vi "Full DMM Scan PRD 32 - 2 SCANs.vi"() -> ()   [LabVIEW 2021]
uses:
  DMM SCAN PRD 32V-16C/Typedefs/Scan configuration.ctl
  <instrlib>/niDMM/nidmm.llb/niDMM Resolution in Digits.ctl
  DMM SCAN PRD 32V-16C/Typedefs/Formatted measurement.ctl
  DMM SCAN PRD 32V-16C/Typedefs/Measurement values.ctl
  DMM Mixed Measurements/DMM Mixed Meas Typedefs/DMM Execution Settings.ctl
  DMM SCAN PRD 32V-16C/Typedefs/Scan Resource Names.ctl
  <instrlib>/niDMM/nidmm.llb/niDMM Powerline Frequency.ctl
  DMM SCAN PRD 32V-16C/Typedefs/Topology.ctl
  <instrlib>/niSwitch/niSwitch.llb/niSwitch Topologies.ctl
  DMM SCAN PRD 32V-16C/Typedefs/Switches Characteristics.ctl
  Static Digital Path Generation/Typedefs/Module Characteristics.ctl
  DMM SCAN PRD 32V-16C/DMM_Scan PXI RLY Driver 32V-16C.lvlib
  DMM Mixed Measurements/DMM_Mixed Measurement.lvlib
  Static Digital Path Generation/Switch_Static Digital Path Generation.lvlib
panel:
  out "Formatted Measurements 2":T1[](array[typedef])=[{"Channel"="ch1", "Switch Time"=0.03192880000005971, "Formatted Measurement"="97.3557mV (dc)", "Out of Range"=FALSE}, {"Channel"="ch32", "Switch Time"=0.040970100000095044, "Formatted Measurement"="9.43379uA (dc)", "Out of Range"=FALSE}, {"Channel"="ch0", "Switch Time"=0.030952699999943434, "Formatted Measurement"="9.89506V (dc)", "Out of Range"=FALSE}] {"Switch Time" format="%#_3p"}
  in  "Scan configuration 2":T2[](array[typedef])=[{"Channel"="ch1", "Resolution in Digits"=5.5, "Range and Function"=enum."DC 100 mV"}, {"Channel"="ch32", "Resolution in Digits"=5.5, "Range and Function"=enum."DC 10 uA"}, {"Channel"="ch0", "Resolution in Digits"=5.5, "Range and Function"=enum."DC 10 V"}] {"Resolution in Digits" items=["3 1/2"=3.5, "4 1/2"=4.5, "5 1/2"=5.5, "6 1/2"=6.5, "7 1/2"=7.5]}
  out "Total Scan Time (s) 2":dbl=0.10385570000016742 format="%#.3p"
  out "Switches Characteristics":T4
  in  "error in":errorcluster
  in  "Relays Debounce Time (ms)":u32=5
  in  "Close all Shunts?":bool=TRUE
  in  "Topology":T6={"MUX Topology Name"="2567/Independent"}
  in  "Powerline Frequency":T8=enum."50 Hz"
  in  "Scan Resources Names":T9={"DMM Resource Name"="DMM_4065", "MUX and Shunt Resource Name"="MUX_2567"}
  out "Total Scan Time (s)":dbl=0.22173839999982192 format="%#.3p"
  out "Execution Settings":T10[](array[typedef])=[{"Absolute\nResolution"=-1e-05, "Input Resistance\n(Ohm)"=10000000.0, "Digits\nResolution"=5.5, "Range"=-1.0, "Minimum\nFrequency (Hz)"=20.0, "Aperture\nTime (s)"=0.003333333333333333, "Auto Range\nValue"=10.0, "Settle\nTime (s)"=-1.0, "Function"=1}, {"Absolute\nResolution"=-1e-05, "Input Resistance\n(Ohm)"=10000000.0, "Digits\nResolution"=5.5, "Range"=-1.0, "Minimum\nFrequency (Hz)"=20.0, "Aperture\nTime (s)"=0.003333333333333333, "Auto Range\nValue"=0.1, "Settle\nTime (s)"=-1.0, "Function"=1}, {"Absolute\nResolution"=-1e-05, "Input Resistance\n(Ohm)"=-1.0, "Digits\nResolution"=5.5, "Range"=-1.0, "Minimum\nFrequency (Hz)"=20.0, "Aperture\nTime (s)"=0.003333333333333333, "Auto Range\nValue"=0.01, "Settle\nTime (s)"=-1.0, "Function"=3}] {"Function" items=["DC Volts"=1, "AC Volts"=2, "DC Current"=3, "AC Current"=4, "2-Wire Resistance"=5, "4-Wire Resistance"=101, "Frequency"=104, "Period"=105, "AC Volts DC Coupled"=1001, "Diode"=1002, "Waveform Voltage"=1003, "Waveform Current"=1004, "Capacitance"=1005, "Inductance"=1006, "Temperature"=108]; "Absolute\nResolution" format="%#_6p"; "Input Resistance\n(Ohm)" format="%#_6p"; "Range" format="%#_6p"; "Minimum\nFrequency (Hz)" format="%#_6p"; "Aperture\nTime (s)" format="%#_6p"; "Auto Range\nValue" format="%#_6p"; "Settle\nTime (s)" format="%#_6p"}
  out "Raw Measurements":T11[](array[typedef])=[{"Channel"="ch0", "Value"=9.895243648852299, "Unit"="V (dc)", "Out of Range"=FALSE}, {"Channel"="ch1", "Value"=0.09675715396605984, "Unit"="V (dc)", "Out of Range"=FALSE}, {"Channel"="ch32", "Value"=9.254776523629187e-06, "Unit"="A (dc)", "Out of Range"=FALSE}] {"Value" format="%#_8g"}
  out "Formatted Measurements":T1[](array[typedef])=[{"Channel"="ch0", "Switch Time"=0.0667068999998719, "Formatted Measurement"="9.89524V (dc)", "Out of Range"=FALSE}, {"Channel"="ch1", "Switch Time"=0.06603180000001885, "Formatted Measurement"="96.7572mV (dc)", "Out of Range"=FALSE}, {"Channel"="ch32", "Switch Time"=0.08899350000001505, "Formatted Measurement"="9.25478uA (dc)", "Out of Range"=FALSE}] {"Switch Time" format="%#_3p"}
  in  "Scan configuration":T2[](array[typedef])=[{"Channel"="ch0", "Resolution in Digits"=5.5, "Range and Function"=enum."DC Voltage Auto Range"}, {"Channel"="ch1", "Resolution in Digits"=5.5, "Range and Function"=enum."DC Voltage Auto Range"}, {"Channel"="ch32", "Resolution in Digits"=5.5, "Range and Function"=enum."DC Current Auto Range"}] {"Resolution in Digits" items=["3 1/2"=3.5, "4 1/2"=4.5, "5 1/2"=5.5, "6 1/2"=6.5, "7 1/2"=7.5]}
  out "error out":errorcluster
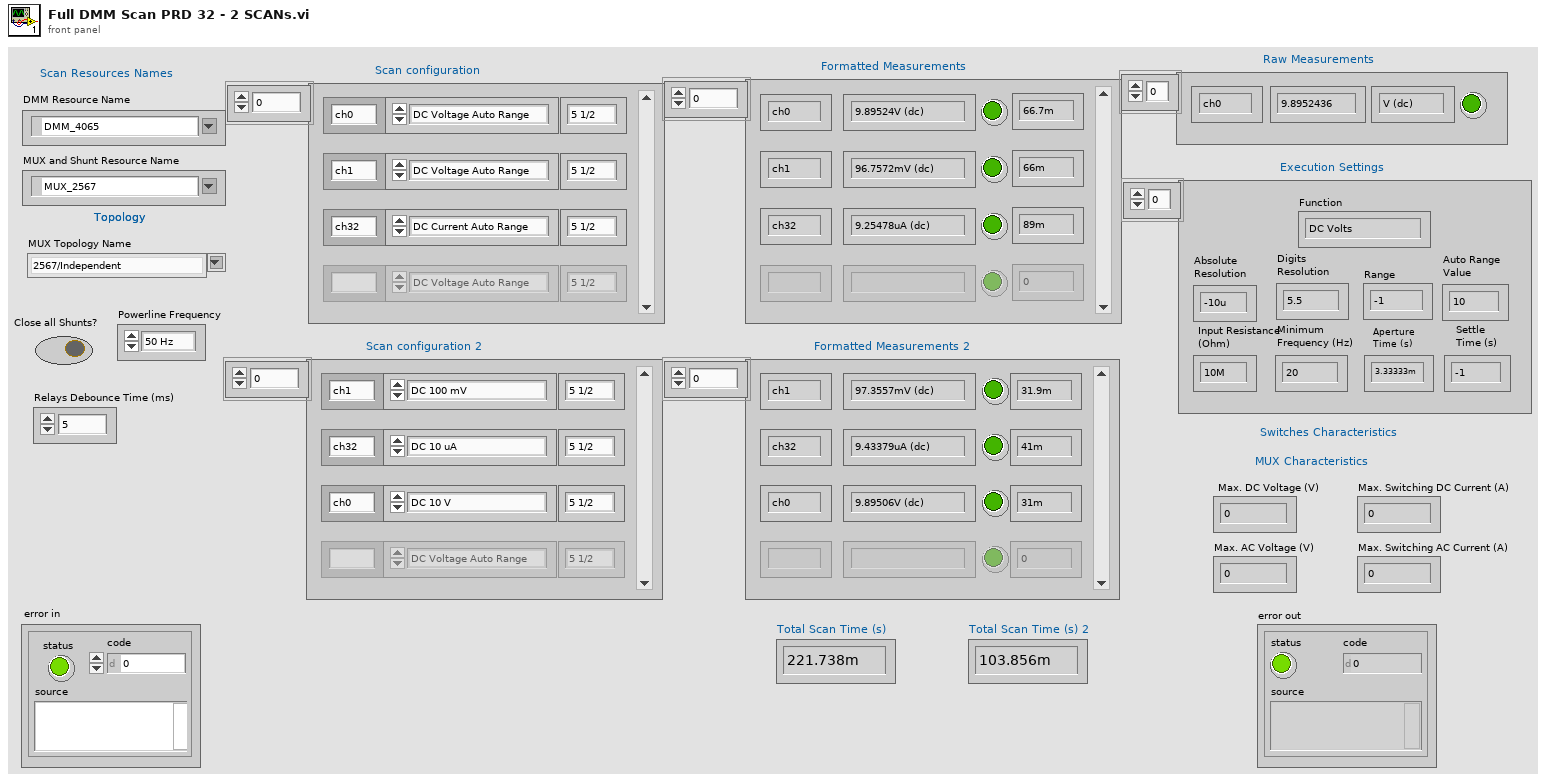
[diagram p1: front panel]
types:
  T1 = typedef "DMM_Scan PXI RLY Driver 32V-16C.lvlib/Formatted measurement.ctl" = cluster{"Channel":string, "Switch Time":dbl, "Formatted Measurement":string, "Out of Range":bool}
  T2 = typedef "DMM_Scan PXI RLY Driver 32V-16C.lvlib/Scan configuration.ctl" = cluster{"Channel":string, "Resolution in Digits":T3, "Range and Function":enum16{"DC Voltage Auto Range", "DC 100 mV", "DC 1 V ", "DC 10 V", "DC 100 V", "DC 300 V", " ", "AC Voltage Auto Range", "AC 50 mV", "AC 200 mV", "AC 500 mV", "AC 2 V", "AC 5 V", "AC 20 V", "AC 50 V", "AC 300 V", "  ", "DC Current Auto Range", "DC 1 uA", "DC 10 uA", "DC 100 uA", "DC 1 mA", "DC 10 mA", "DC 20 mA", "DC 100 mA", "DC 200 mA", "DC 1 A", "DC 3 A", "   ", "AC Current Auto Range", "AC 100 uA", "AC 1 mA", "AC 10 mA", "AC 100 mA", "AC 500 mA", "AC 1 A", "AC 3 A", "    ", "Resistance Auto Range", "Res 100 Ohm", "Res 1 kOhm", "Res 10 kOhm", "Res 100 kOhm", "Res 1 MOhm", "Res 10 MOhm", "Res 100 MOhm", "Res 5 GOhm", "     ", "Frequency AC Auto Range", "Freq AC 50 mV", "Freq AC 500 mV", "Freq AC 5 V", "Freq AC 50 V", "Freq AC 300 V", "      ", "Period AC Auto Range", "Period AC 50 mV", "Period AC 500 mV", "Period AC 5 V", "Period AC 50 V", "Period AC 300 V"}}
  T3 = typedef "niDMM Resolution in Digits.ctl" = dbl
  T4 = typedef "DMM_Scan PXI RLY Driver 32V-16C.lvlib/Switches Characteristics.ctl" = cluster{"Mux Characteristics":T5}
  T5 = typedef "Switch_Static Digital Path Generation.lvlib/Module Characteristics.ctl" = cluster{" Max. DC Voltage (V)":dbl, "Max. Switching DC Current (A)":dbl, "Max. AC Voltage (V)":dbl, "Max. Switching AC Current (A)":dbl}
  T6 = typedef "DMM_Scan PXI RLY Driver 32V-16C.lvlib/Topology.ctl" = cluster{"MUX Topology Name":T7}
  T7 = typedef "niSwitch Topologies.ctl" = string
  T8 = typedef "niDMM Powerline Frequency.ctl" = enum16{"60 Hz", "50 Hz"}
  T9 = typedef "DMM_Scan PXI RLY Driver 32V-16C.lvlib/Scan Resource Names.ctl" = cluster{"DMM Resource Name":refnum<k15>, "MUX and Shunt Resource Name":refnum<k15>}
  T10 = typedef "DMM_Mixed Measurement.lvlib/DMM Execution Settings.ctl" = cluster{"Absolute\nResolution":dbl, "Input Resistance\n(Ohm)":dbl, "Digits\nResolution":dbl, "Range":dbl, "Minimum\nFrequency (Hz)":dbl, "Aperture\nTime (s)":dbl, "Auto Range\nValue":dbl, "Settle\nTime (s)":dbl, "Function":i32}
  T11 = typedef "DMM_Scan PXI RLY Driver 32V-16C.lvlib/Measurement values.ctl" = cluster{"Channel":string, "Value":dbl, "Unit":string, "Out of Range":bool}
  T12 = typedef "DMM_Scan PXI RLY Driver 32V-16C.lvlib/Scan Resource Handles Out.ctl" = cluster{"DMM Handle":refnum<k15>, "MUX Handle":refnum<k15>, "Relays Debounce Time (ms)":u32, "Close all Shunts?":bool}
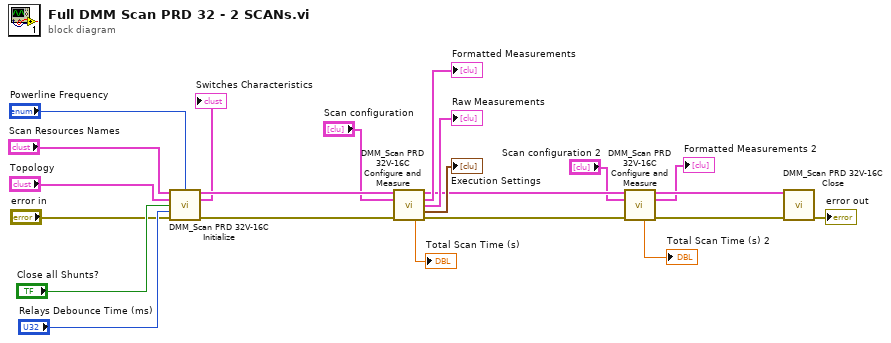
[diagram p0: block diagram]
diagram:
  n1 = call "DMM_Scan PRD 32V-16C Initialize.vi"("Scan Resource Names"="Scan Resources Names", "Powerline Frequency"="Powerline Frequency", "Topology"="Topology", "Close all Shunts?"="Close all Shunts?", "Relay Debounce Time (ms)"="Relays Debounce Time (ms)", "error in"="error in") -> ("Scan Resource Handles out"=w21:T12, "Switches Characteristics"=→"Switches Characteristics":T4, "error out"=w22:errorcluster)  [unwired: 7 in]
  n2 = call "DMM_Scan PRD 32V-16C Configure and Measure.vi"("Scan Resources Handles In"=w21, "Scan Configuration"="Scan configuration", "error in"=w22) -> ("Scan Resources Handles Out"=w4:T12, "Formatted Measurements"=→"Formatted Measurements":T1[], "Raw Measurements"=→"Raw Measurements":T11[], "Execution Settings"=→"Execution Settings":T10[], "Total Scan Time (s)"=→"Total Scan Time (s)":dbl, "error out"=w7:errorcluster)  [unwired: 7 in]
  n3 = call "DMM_Scan PRD 32V-16C Configure and Measure.vi"("Scan Resources Handles In"=w4, "Scan Configuration"="Scan configuration 2", "error in"=w7) -> ("Scan Resources Handles Out"=w3:T12, "Formatted Measurements"=→"Formatted Measurements 2":T1[], "Total Scan Time (s)"=→"Total Scan Time (s) 2":dbl, "error out"=w6:errorcluster)  [unwired: 7 in, 2 out]
  n4 = call "DMM_Scan PRD 32V-16C Close.vi"("Scan Resources Handles In"=w3, "error in"=w6) -> ("error out"=→"error out":errorcluster)  [unwired: 13 in]
